vi "PH_Switch.ProcCases.vi"(0 "i ref in":refnum<vi>, 1 "selector":string, 2 "Data":T1, 3 "call cluster":T2={"Object"="", "Selector"="", "CallType"=enum."synchronous", "Async Object"="", "Async Selector"="", "Data Descriptor"="", "Data"=[], "Error #"=0, "Expire"=0}, 5 "error in (no error)":errorcluster) -> (14 "i ref out":refnum<vi>, 17 "answer cluster":T2={"Object"="", "Selector"="", "CallType"=enum."synchronous", "Async Object"="", "Async Selector"="", "Data Descriptor"="", "Data"=[], "Error #"=0, "Expire"=0}, 19 "error out":errorcluster)   [LabVIEW 2014, in "PH_Switch.lvlib"]
doc: "This method is called by a process from within the default case in the event loop. The methods of a class that are linked to events will be called from THIS method. Add your code here."
uses:
  PH_Switch.lvlib
  CSCore/CSSystem/CoreDefs/CoreDefs.call_type.ctl
  CSCore/BaseProcess/BaseProcess.descriptor string definition.ctl
  CSCore/CSSystem/CoreDefs/CoreDefs.rawDataType.ctl
  PH_StatusHandler/PH_StatusHandler.Status.ctl
  CSCore/CSSystem/CoreLib/CoreLib.string 2 byte array.vi
  CSCore/CSSystem/CoreLib/CoreLib.byte array 2 short.vi
  CSCore/CSSystem/CoreLib/CoreLib.byte array 2 string.vi
  PH_Common/PH_Common.lvlib
  CSCore/CSSystem/CoreLib/CoreLib.lvlib
  CSCore/BaseProcess/BaseProcess.lvlib
  CSCore/CAEObj/CAEObj.lvlib
  PH_Sixpack_Switch/PH_Sixpack_Switch.lvlib
  PH_PSDBWriter/PH_PSDBWriter.lvlib
  PH_StatusHandler/PH_StatusHandler.lvlib
  PH_Beckhoff/PH_Beckhoff.lvlib
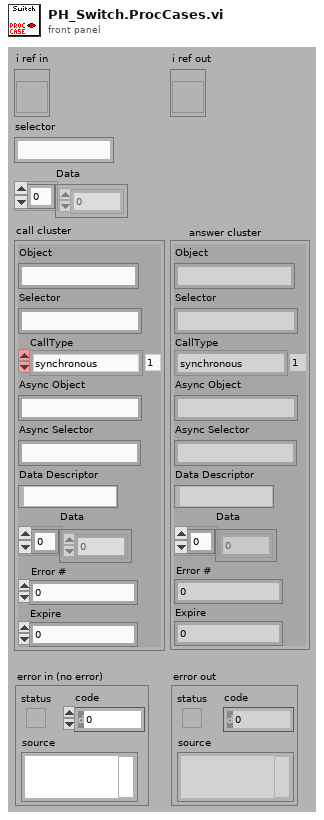
[diagram p1: front panel]
types:
  T1 = typedef "CoreDefs.rawDataType.ctl" = i8[]
  T2 = typedef "CoreDefs.call_type.ctl" = cluster{"Object":string, "Selector":string, "CallType":enum16{"simple", "synchronous", "asynchronous"}, "Async Object":string, "Async Selector":string, "Data Descriptor":T3, "Data":T1, "Error #":i32, "Expire":u32}
  T3 = typedef "BaseProcess.lvlib/BaseProcess.descriptor string definition.ctl" = string
  T4 = typedef "PH_Switch.lvlib/PH_Switch.i attribute.ctl" = cluster{"GUI Refs":T5, "Status true":T6, "Status false":T6, "Status Switch State":T6, "remote controlled":bool, "Tagname":cluster{"Switch":string, "True":string, "False":string}, "Beckhoff Instance":string, "Caption":cluster{"True":string, "False":string}, "Default State":string}
  T5 = typedef "PH_Switch.lvlib/PH_Switch.GUI Refs.ctl" = cluster{"true":refnum<vi>, "false":refnum<vi>, "Switch_state":refnum<vi>, "GUI-Knob":refnum<vi>, "Delete":refnum<vi>, "Function Textfield":refnum<vi>}
  T6 = typedef "PH_StatusHandler.lvlib/PH_StatusHandler.Status.ctl" = i16
  T7 = typedef "PH_PSDBWriter.lvlib/PH_PSDBWriter.PHELIX-Subsystems.ctl" = i32
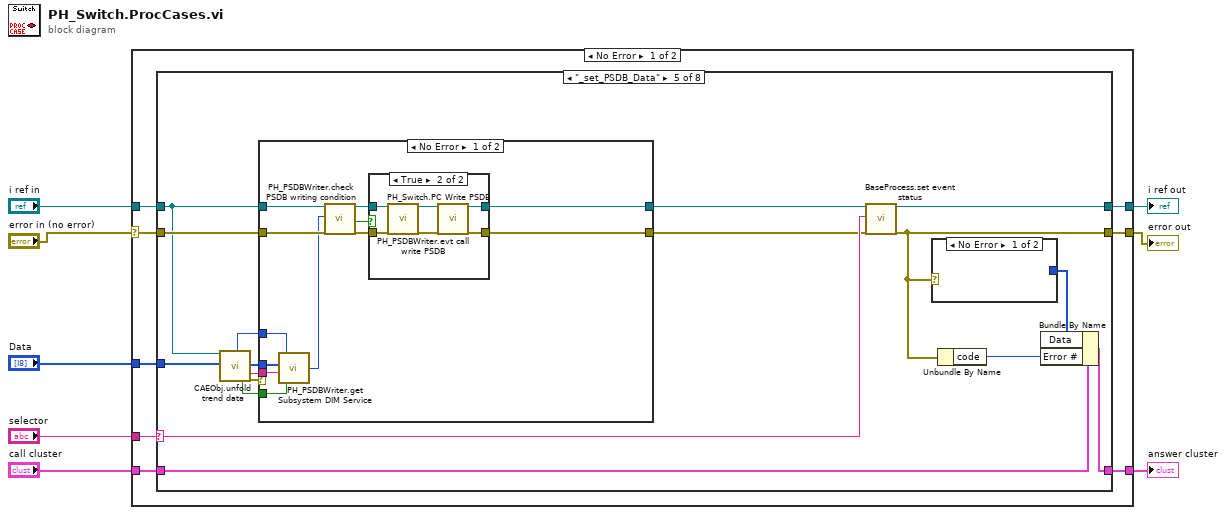
[diagram p0: block diagram]
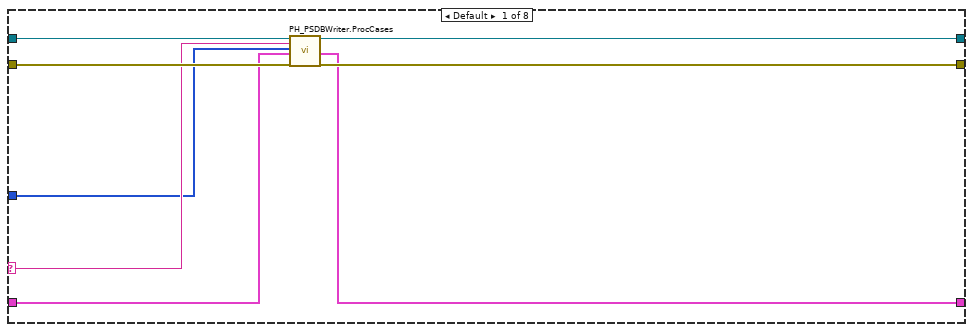
[diagram p2: hidden frame]
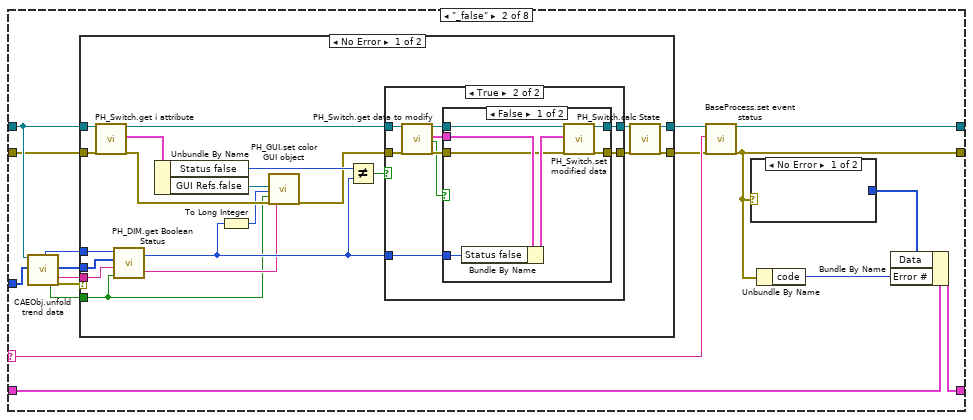
[diagram p3: hidden frame]
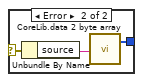
[diagram p7: hidden frame]
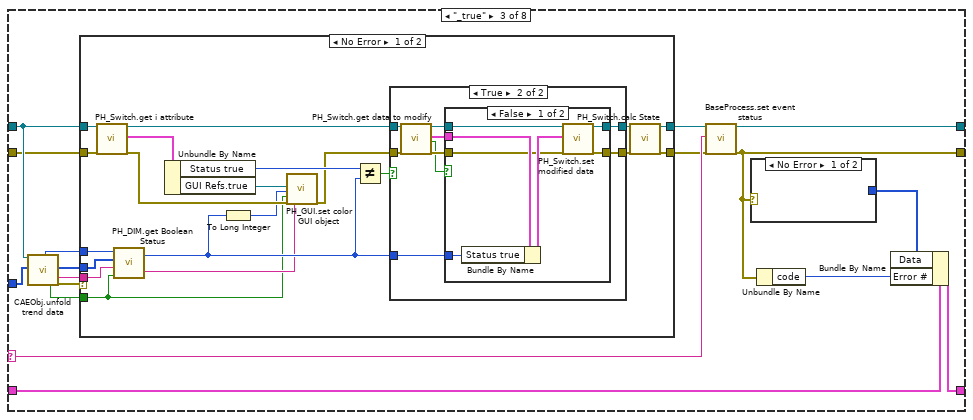
[diagram p8: hidden frame]
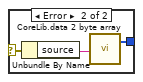
[diagram p12: hidden frame]
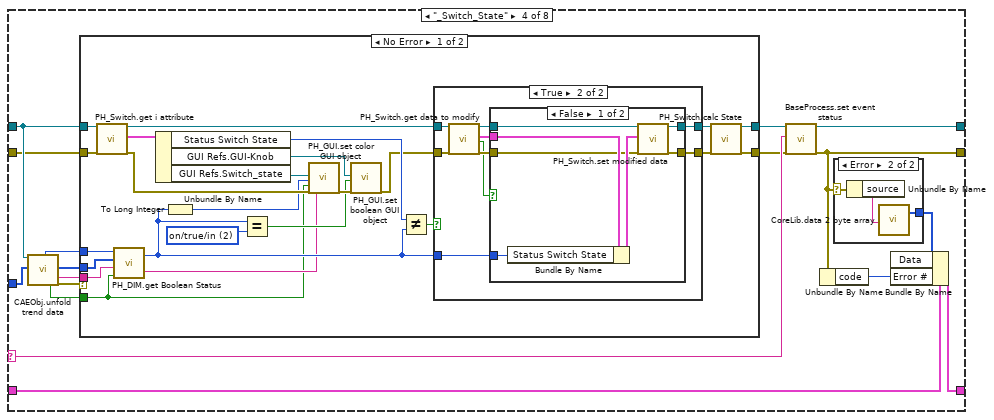
[diagram p13: hidden frame]
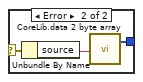
[diagram p20: hidden frame]
diagram:
  n1 = case shown="No Error" "error in (no error)" {
    selector: "error in (no error)" -> [w9 w383]
    tunnel: "selector" -> [w16 _]
    tunnel: [w15 w382] -> w7
    tunnel: "call cluster" -> [w14 w382]
    tunnel: "i ref in" -> [w13 w384]
    tunnel: [w12 w384] -> w5
    tunnel: [w11 w383] -> w4
    tunnel: "Data" -> [w10 _]
    frame No Error {
      n2 = case shown="\"_set_PSDB_Data\"" w16 {
        selector: w16 -> [w19 w39 w101 w163 w225 w261 w310 w353]
        tunnel: w13 -> [w18 w33 w95 w157 w216 w270 w314 w357]
        tunnel: [w24 w37 w99 w161 w228 w257 w312 w355] -> w12
        tunnel: w14 -> [w20 w35 w97 w159 w227 w260 w309 w352]
        tunnel: [w21 w34 w96 w158 w226 w259 w308 w351] -> w15
        tunnel: w9 -> [w23 w32 w94 w156 w219 w271 w313 w356]
        tunnel: [w22 w36 w98 w160 w229 w258 w311 w354] -> w11
        tunnel: w10 -> [w17 w38 w100 w162 w215 _ _ _]
        frame Default {
          n3 = call "PH_PSDBWriter.ProcCases.vi"("i ref in"=w18, "selector"=w19, "Data"=w17, "call cluster"=w20, "error in"=w23) -> ("i ref out"=w24:refnum<vi>, "answer cluster"=w21:T2, "error out"=w22:errorcluster)  [unwired: 12 in]
        }
        frame "_false" {
          n4 = call "CAEObj.unfold trend data.vi"("i ref in"=w33, "raw trend data"=w38) -> ("quality"=w26:i32, "no link"=w28:bool, "data"=w27:i8[], "typeDescriptor"=w25:string, "error out"=w29:errorcluster)  [unwired: 9 in, 4 out]
          n5 = case shown="No Error" w29 {
            tunnel: w32 -> [w61 w82]
            tunnel: [w52 w83] -> w30
            tunnel: [w50 w82] -> w31
            tunnel: w33 -> [w57 w83]
            tunnel: w28 -> [w42 _]
            tunnel: w25 -> [w60 _]
            tunnel: w27 -> [w58 _]
            tunnel: w26 -> [w59 _]
            frame No Error {
              n6 = call "PH_Switch.get i attribute.vi"("i ref in"=w57, "error in (no error)"=w61) -> ("i ref out"=w56:refnum<vi>, "i attribute"=w55:T4, "error out"=w47:errorcluster)  [unwired: 15 in]
              n7 = call "PH_DIM.get Boolean Status.vi"("no link"=w42, "typeDescriptor"=w60, "data"=w58, "quality"=w59) -> ("further information"=w44:string, "Status"=w45:T6)
              n8 = Unbundle By Name(w55) -> ("Status false"=w54:T6, "GUI Refs.false"=w48:refnum<vi>)
              n9 = To Long Integer(number=w45) -> (32bit integer=w43:i32)
              n10 = call "PH_GUI.set color GUI object.vi"("GUI object Ref"=w48, "State"=w43, "Blinking? (false)"=w42, "error in (no error)"=w47, "Tip Strip (N/A)"=w44) -> ("error out"=w46:errorcluster)  [unwired: 14 in]
              n11 = Not Equal?(x=w54, y=w45) -> (x != y?=w53:bool)
              n12 = case shown="True" w53 {
                tunnel: [w63 w65] -> w51
                tunnel: [w62 w64] -> w49
                tunnel: w46 -> [w62 w68]
                tunnel: w56 -> [w63 w67]
                tunnel: w45 -> [_ w66]
                frame False {
                }
                frame True {
                  n13 = call "PH_Switch.get data to modify.vi"("i ref in"=w67, "error in (no error)"=w68) -> ("i ref out"=w71:refnum<vi>, "i attribute"=w70:T4, "timed out"=w69:bool, "error out"=w72:errorcluster)  [unwired: 14 in]
                  n14 = case shown="False" w69 {
                    tunnel: w72 -> [w73 w81]
                    tunnel: [w79 w81] -> w64
                    tunnel: [w78 w80] -> w65
                    tunnel: w71 -> [w74 w80]
                    tunnel: w70 -> [w77 _]
                    tunnel: w66 -> [w75 _]
                    frame False {
                      n15 = Bundle By Name(cluster=w77, "Status false"=w75) -> (w76:T4)
                      n16 = call "PH_Switch.set modified data.vi"("i ref in"=w74, "i attribute"=w76, "error in (no error)"=w73) -> ("i ref out"=w78:refnum<vi>, "error out"=w79:errorcluster)  [unwired: 15 in]
                    }
                    frame True {
                    }
                  }
                }
              }
              n17 = call "PH_Switch.calc State.vi"("i ref in"=w51, "error in (no error)"=w49) -> ("i ref out"=w52:refnum<vi>, "error out"=w50:errorcluster)  [unwired: 16 in]
            }
            frame Error {
            }
          }
          n18 = call "BaseProcess.set event status.vi"("i ref in"=w30, "EventStatus"=w39, "error in (no error)"=w31) -> ("i ref out"=w37:refnum<vi>, "error out"=w36:errorcluster)  [unwired: 14 in, 1 out]
          n19 = case shown="No Error" w36 {
            selector: w36 -> [_ w86]
            tunnel: [_ w84] -> w41
            frame No Error {
            }
            frame Error {
              n20 = Unbundle By Name(w86) -> ("source"=w85:string)
              n21 = call-poly "CoreLib.data 2 byte array.vi"("string"=w85) -> ("byteArray out"=w84:T1)  [unwired: 18 in]
            }
          }
          n22 = Unbundle By Name(w36) -> ("code"=w40:i32)
          n23 = Bundle By Name(cluster=w35, "Data"=w41, "Error #"=w40) -> (w34:T2)
        }
        frame "_true" {
          n24 = call "CAEObj.unfold trend data.vi"("i ref in"=w95, "raw trend data"=w100) -> ("quality"=w88:i32, "no link"=w90:bool, "data"=w89:i8[], "typeDescriptor"=w87:string, "error out"=w91:errorcluster)  [unwired: 9 in, 4 out]
          n25 = case shown="No Error" w91 {
            tunnel: w94 -> [w123 w144]
            tunnel: [w113 w145] -> w92
            tunnel: [w111 w144] -> w93
            tunnel: w95 -> [w119 w145]
            tunnel: w90 -> [w104 _]
            tunnel: w87 -> [w122 _]
            tunnel: w89 -> [w120 _]
            tunnel: w88 -> [w121 _]
            frame No Error {
              n26 = call "PH_Switch.get i attribute.vi"("i ref in"=w119, "error in (no error)"=w123) -> ("i ref out"=w118:refnum<vi>, "i attribute"=w117:T4, "error out"=w109:errorcluster)  [unwired: 15 in]
              n27 = call "PH_DIM.get Boolean Status.vi"("no link"=w104, "typeDescriptor"=w122, "data"=w120, "quality"=w121) -> ("further information"=w105:string, "Status"=w107:T6)
              n28 = Unbundle By Name(w117) -> ("Status true"=w116:T6, "GUI Refs.true"=w110:refnum<vi>)
              n29 = To Long Integer(number=w107) -> (32bit integer=w106:i32)
              n30 = call "PH_GUI.set color GUI object.vi"("GUI object Ref"=w110, "State"=w106, "Blinking? (false)"=w104, "error in (no error)"=w109, "Tip Strip (N/A)"=w105) -> ("error out"=w108:errorcluster)  [unwired: 14 in]
              n31 = Not Equal?(x=w116, y=w107) -> (x != y?=w115:bool)
              n32 = case shown="True" w115 {
                tunnel: [w125 w127] -> w112
                tunnel: [w124 w126] -> w114
                tunnel: w108 -> [w124 w130]
                tunnel: w118 -> [w125 w129]
                tunnel: w107 -> [_ w128]
                frame False {
                }
                frame True {
                  n33 = call "PH_Switch.get data to modify.vi"("i ref in"=w129, "error in (no error)"=w130) -> ("i ref out"=w133:refnum<vi>, "i attribute"=w132:T4, "timed out"=w131:bool, "error out"=w134:errorcluster)  [unwired: 14 in]
                  n34 = case shown="False" w131 {
                    tunnel: w134 -> [w135 w143]
                    tunnel: [w141 w143] -> w126
                    tunnel: [w140 w142] -> w127
                    tunnel: w133 -> [w136 w142]
                    tunnel: w132 -> [w139 _]
                    tunnel: w128 -> [w137 _]
                    frame False {
                      n35 = Bundle By Name(cluster=w139, "Status true"=w137) -> (w138:T4)
                      n36 = call "PH_Switch.set modified data.vi"("i ref in"=w136, "i attribute"=w138, "error in (no error)"=w135) -> ("i ref out"=w140:refnum<vi>, "error out"=w141:errorcluster)  [unwired: 15 in]
                    }
                    frame True {
                    }
                  }
                }
              }
              n37 = call "PH_Switch.calc State.vi"("i ref in"=w112, "error in (no error)"=w114) -> ("i ref out"=w113:refnum<vi>, "error out"=w111:errorcluster)  [unwired: 16 in]
            }
            frame Error {
            }
          }
          n38 = call "BaseProcess.set event status.vi"("i ref in"=w92, "EventStatus"=w101, "error in (no error)"=w93) -> ("i ref out"=w99:refnum<vi>, "error out"=w98:errorcluster)  [unwired: 14 in, 1 out]
          n39 = case shown="No Error" w98 {
            selector: w98 -> [_ w148]
            tunnel: [_ w146] -> w103
            frame No Error {
            }
            frame Error {
              n40 = Unbundle By Name(w148) -> ("source"=w147:string)
              n41 = call-poly "CoreLib.data 2 byte array.vi"("string"=w147) -> ("byteArray out"=w146:T1)  [unwired: 18 in]
            }
          }
          n42 = Unbundle By Name(w98) -> ("code"=w102:i32)
          n43 = Bundle By Name(cluster=w97, "Data"=w103, "Error #"=w102) -> (w96:T2)
        }
        frame "_Switch_State" {
          n44 = call "CAEObj.unfold trend data.vi"("i ref in"=w157, "raw trend data"=w162) -> ("quality"=w150:i32, "no link"=w152:bool, "data"=w151:i8[], "typeDescriptor"=w149:string, "error out"=w153:errorcluster)  [unwired: 9 in, 4 out]
          n45 = case shown="No Error" w153 {
            tunnel: w156 -> [w189 w210]
            tunnel: [w178 w211] -> w154
            tunnel: [w177 w210] -> w155
            tunnel: w157 -> [w185 w211]
            tunnel: w152 -> [w166 _]
            tunnel: w149 -> [w188 _]
            tunnel: w151 -> [w186 _]
            tunnel: w150 -> [w187 _]
            frame No Error {
              w168 = T6 2 items=["no info", "off/false/out", "on/true/in", "Failure", "Alarm", "Status 1", "Status 2", "Status 3"] ("y")
              n46 = call "PH_Switch.get i attribute.vi"("i ref in"=w185, "error in (no error)"=w189) -> ("i ref out"=w184:refnum<vi>, "i attribute"=w183:T4, "error out"=w175:errorcluster)  [unwired: 15 in]
              n47 = call "PH_DIM.get Boolean Status.vi"("no link"=w166, "typeDescriptor"=w188, "data"=w186, "quality"=w187) -> ("further information"=w167:string, "Status"=w170:T6)
              n48 = Unbundle By Name(w183) -> ("Status Switch State"=w182:T6, "GUI Refs.GUI-Knob"=w172:refnum<vi>, "GUI Refs.Switch_state"=w173:refnum<vi>)
              n49 = To Long Integer(number=w170) -> (32bit integer=w169:i32)
              n50 = Equal?(x=w170, y=w168) -> (x = y?=w171:bool)
              n51 = call "PH_GUI.set color GUI object.vi"("GUI object Ref"=w173, "State"=w169, "Blinking? (false)"=w166, "error in (no error)"=w175, "Tip Strip (N/A)"=w167) -> ("error out"=w176:errorcluster)  [unwired: 14 in]
              n52 = call "PH_GUI.set boolean GUI object.vi"("Boolean Knob GUI Ref"=w172, "Value"=w171, "error in (no error)"=w176) -> ("error out"=w174:errorcluster)  [unwired: 16 in]
              n53 = Not Equal?(x=w182, y=w170) -> (x != y?=w181:bool)
              n54 = case shown="True" w181 {
                tunnel: [w191 w193] -> w180
                tunnel: [w190 w192] -> w179
                tunnel: w174 -> [w190 w196]
                tunnel: w184 -> [w191 w195]
                tunnel: w170 -> [_ w194]
                frame False {
                }
                frame True {
                  n55 = call "PH_Switch.get data to modify.vi"("i ref in"=w195, "error in (no error)"=w196) -> ("i ref out"=w199:refnum<vi>, "i attribute"=w198:T4, "timed out"=w197:bool, "error out"=w200:errorcluster)  [unwired: 14 in]
                  n56 = case shown="False" w197 {
                    tunnel: w200 -> [w201 w209]
                    tunnel: [w207 w209] -> w192
                    tunnel: [w206 w208] -> w193
                    tunnel: w199 -> [w203 w208]
                    tunnel: w198 -> [w205 _]
                    tunnel: w194 -> [w202 _]
                    frame False {
                      n57 = Bundle By Name(cluster=w205, "Status Switch State"=w202) -> (w204:T4)
                      n58 = call "PH_Switch.set modified data.vi"("i ref in"=w203, "i attribute"=w204, "error in (no error)"=w201) -> ("i ref out"=w206:refnum<vi>, "error out"=w207:errorcluster)  [unwired: 15 in]
                    }
                    frame True {
                    }
                  }
                }
              }
              n59 = call "PH_Switch.calc State.vi"("i ref in"=w180, "error in (no error)"=w179) -> ("i ref out"=w178:refnum<vi>, "error out"=w177:errorcluster)  [unwired: 16 in]
            }
            frame Error {
            }
          }
          n60 = call "BaseProcess.set event status.vi"("i ref in"=w154, "EventStatus"=w163, "error in (no error)"=w155) -> ("i ref out"=w161:refnum<vi>, "error out"=w160:errorcluster)  [unwired: 14 in, 1 out]
          n61 = Unbundle By Name(w160) -> ("code"=w164:i32)
          n62 = case shown="Error" w160 {
            selector: w160 -> [_ w214]
            tunnel: [_ w212] -> w165
            frame No Error {
            }
            frame Error {
              n63 = Unbundle By Name(w214) -> ("source"=w213:string)
              n64 = call-poly "CoreLib.data 2 byte array.vi"("string"=w213) -> ("byteArray out"=w212:T1)  [unwired: 18 in]
            }
          }
          n65 = Bundle By Name(cluster=w159, "Data"=w165, "Error #"=w164) -> (w158:T2)
        }
        frame "_set_PSDB_Data" {
          n66 = call "CAEObj.unfold trend data.vi"("i ref in"=w216, "raw trend data"=w215) -> ("quality"=w222:i32, "no link"=w221:bool, "data"=w224:i8[], "typeDescriptor"=w223:string, "error out"=w220:errorcluster)  [unwired: 9 in, 4 out]
          n67 = case shown="No Error" w220 {
            tunnel: w219 -> [w243 w253]
            tunnel: [w242 w252] -> w218
            tunnel: [w241 w253] -> w217
            tunnel: w216 -> [w235 w252]
            tunnel: w221 -> [w240 _]
            tunnel: w223 -> [w239 _]
            tunnel: w224 -> [w238 _]
            tunnel: w222 -> [w237 _]
            frame No Error {
              n68 = call "PH_PSDBWriter.get Subsystem DIM Service.vi"("no link"=w240, "typeDescriptor"=w239, "data"=w238, "quality"=w237) -> ("PHELIX Subsystems"=w232:T7)
              n69 = call "PH_PSDBWriter.check PSDB writing condition.vi"("i ref in"=w235, "wanted Subsystem"=w232, "error IO"=w243) -> ("i ref out"=w234:refnum<vi>, "write PSDB?"=w233:bool, "error out"=w236:errorcluster)  [unwired: 14 in]
              n70 = case shown="True" w233 {
                tunnel: w236 -> [w244 w251]
                tunnel: [w245 w246] -> w242
                tunnel: [w244 w247] -> w241
                tunnel: w234 -> [w245 w250]
                frame False {
                }
                frame True {
                  n71 = call "PH_Switch.PC Write PSDB.vi"("i ref in"=w250, "error IO"=w251) -> ("i ref out"=w249:refnum<vi>, "error out"=w248:errorcluster)  [unwired: 16 in]
                  n72 = call "PH_PSDBWriter.evt call write PSDB.vi"("i ref in"=w249, "error in (no error)"=w248) -> ("i ref out"=w246:refnum<vi>, "error out"=w247:errorcluster)  [unwired: 16 in]
                }
              }
            }
            frame Error {
            }
          }
          n73 = call "BaseProcess.set event status.vi"("i ref in"=w218, "EventStatus"=w225, "error in (no error)"=w217) -> ("i ref out"=w228:refnum<vi>, "error out"=w229:errorcluster)  [unwired: 14 in, 1 out]
          n74 = case shown="No Error" w229 {
            selector: w229 -> [_ w256]
            tunnel: [_ w254] -> w230
            frame No Error {
            }
            frame Error {
              n75 = Unbundle By Name(w256) -> ("source"=w255:string)
              n76 = call-poly "CoreLib.data 2 byte array.vi"("string"=w255) -> ("byteArray out"=w254:T1)  [unwired: 18 in]
            }
          }
          n77 = Unbundle By Name(w229) -> ("code"=w231:i32)
          n78 = Bundle By Name(cluster=w227, "Data"=w230, "Error #"=w231) -> (w226:T2)
        }
        frame "Switch" {
          n79 = Unbundle By Name(w260) -> ("Data"=w269:T1)
          n80 = call-poly "CoreLib.byte array 2 data.vi"("byteArray"=w269) -> ("i16"=w268:i16, "error out"=w267:errorcluster)  [unwired: 16 in, 1 out]
          n81 = Greater Than 0?(x=w268) -> (x > 0?=w266:bool)
          n82 = case shown="No Error" w267 {
            tunnel: [w284 w307] -> w263
            tunnel: [w283 w304] -> w262
            tunnel: w270 -> [w277 w307]
            tunnel: w271 -> [w276 w306]
            tunnel: w261 -> [_ w305]
            tunnel: w266 -> [w282 _]
            frame No Error {
              n83 = call "PH_Switch.get i attribute.vi"("i ref in"=w277, "error in (no error)"=w276) -> ("i ref out"=w285:refnum<vi>, "i attribute"=w287:T4, "error out"=w286:errorcluster)  [unwired: 15 in]
              n84 = Unbundle By Name(w287) -> ("GUI Refs.GUI-Knob"=w280:refnum<vi>, "Beckhoff Instance"=w278:string, "Tagname.Switch"=w275:string)
              n85 = call "PH_Switch.check 6P Switch.vi"("Tagname"=w275) -> ("Tagname 6P Switch"=w281:string, "6P Switch?"=w279:bool)
              n86 = case shown="False" w279 {
                tunnel: w286 -> [w294 w303]
                tunnel: w285 -> [w296 w302]
                tunnel: [w295 w301] -> w284
                tunnel: [w290 w300] -> w283
                tunnel: w278 -> [_ w299]
                tunnel: w282 -> [w292 w298]
                tunnel: w275 -> [_ w297]
                tunnel: w281 -> [w293 _]
                tunnel: w280 -> [w289 _]
                frame True {
                  n87 = call "PH_Sixpack_Switch.evt move.vi"("i ref in"=w296, "Instance"=w293, "Move"=w292, "error in (no error)"=w294) -> ("i ref out"=w295:refnum<vi>, "error out"=w291:errorcluster)  [unwired: 14 in]
                  n88 = call "PH_GUI.set boolean GUI object.vi"("Boolean Knob GUI Ref"=w289, "Value"=FALSE, "error in (no error)"=w291) -> ("error out"=w290:errorcluster)  [unwired: 16 in]
                }
                frame False {
                  n89 = call "PH_Beckhoff.evt Call Set Boolean Value.vi"("i ref in"=w302, "Beckhoff Instance"=w299, "Tagname to set"=w297, "Value"=w298, "error in"=w303) -> ("i ref out"=w301:refnum<vi>, "error out"=w300:errorcluster)  [unwired: 13 in]
                }
              }
            }
            frame Error {
              n90 = call "CoreLib.set data type mismatch.vi"("error in (no error)"=w306, "error source"=w305) -> ("error out"=w304:errorcluster)  [unwired: 17 in]
            }
          }
          n91 = call "BaseProcess.set event status.vi"("i ref in"=w263, "EventStatus"=w261, "error in (no error)"=w262) -> ("i ref out"=w257:refnum<vi>, "error out"=w258:errorcluster)  [unwired: 14 in, 1 out]
          n92 = Unbundle By Name(w258) -> ("code"=w265:i32)
          n93 = case shown="No Error" w258 {
            selector: w258 -> [_ w274]
            tunnel: [_ w272] -> w264
            frame No Error {
            }
            frame Error {
              n94 = Unbundle By Name(w274) -> ("source"=w273:string)
              n95 = call-poly "CoreLib.data 2 byte array.vi"("string"=w273) -> ("byteArray out"=w272:T1)  [unwired: 18 in]
            }
          }
          n96 = Bundle By Name(cluster=w260, "Data"=w264, "Error #"=w265) -> (w259:T2)
        }
        frame "Control Remote" {
          n97 = Unbundle By Name(w309) -> ("Data"=w317:T1)
          n98 = call-poly "CoreLib.byte array 2 data.vi"("byteArray"=w317) -> ("i16"=w318:i16, "error out"=w320:errorcluster)  [unwired: 16 in, 1 out]
          n99 = Greater Than 0?(x=w318) -> (x > 0?=w319:bool)
          n100 = case shown="No Error" w320 {
            tunnel: [w329 w349] -> w315
            tunnel: w314 -> [w336 w349]
            tunnel: w313 -> [w335 w348]
            tunnel: [w327 w347] -> w316
            tunnel: w310 -> [_ w346]
            tunnel: w319 -> [w333 _]
            frame No Error {
              n101 = call "PH_Switch.get data to modify.vi"("i ref in"=w336, "error in (no error)"=w335) -> ("i ref out"=w331:refnum<vi>, "i attribute"=w332:T4, "timed out"=w330:bool, "error out"=w334:errorcluster)  [unwired: 14 in]
              n102 = case shown="False" w330 {
                tunnel: w334 -> [w343 w345]
                tunnel: [w342 w345] -> w326
                tunnel: w333 -> [w337 _]
                tunnel: w332 -> [w341 _]
                tunnel: w331 -> [w340 w344]
                tunnel: [w339 w344] -> w328
                frame False {
                  n103 = Bundle By Name(cluster=w341, "remote controlled"=w337) -> (w338:T4)
                  n104 = call "PH_Switch.set modified data.vi"("i ref in"=w340, "i attribute"=w338, "error in (no error)"=w343) -> ("i ref out"=w339:refnum<vi>, "error out"=w342:errorcluster)  [unwired: 15 in]
                }
                frame True {
                }
              }
              n105 = call "PH_Switch.calc State.vi"("i ref in"=w328, "error in (no error)"=w326) -> ("i ref out"=w329:refnum<vi>, "error out"=w327:errorcluster)  [unwired: 16 in]
            }
            frame Error {
              n106 = call "CoreLib.set data type mismatch.vi"("error in (no error)"=w348, "error source"=w346) -> ("error out"=w347:errorcluster)  [unwired: 17 in]
            }
          }
          n107 = call "BaseProcess.set event status.vi"("i ref in"=w315, "EventStatus"=w310, "error in (no error)"=w316) -> ("i ref out"=w312:refnum<vi>, "error out"=w311:errorcluster)  [unwired: 14 in, 1 out]
          n108 = case shown="Error" w311 {
            selector: w311 -> [_ w325]
            tunnel: [_ w323] -> w322
            frame No Error {
            }
            frame Error {
              n109 = Unbundle By Name(w325) -> ("source"=w324:string)
              n110 = call-poly "CoreLib.data 2 byte array.vi"("string"=w324) -> ("byteArray out"=w323:T1)  [unwired: 18 in]
            }
          }
          n111 = Unbundle By Name(w311) -> ("code"=w321:i32)
          n112 = Bundle By Name(cluster=w309, "Data"=w322, "Error #"=w321) -> (w308:T2)
        }
        frame "Set Function Textfield" {
          n113 = Unbundle By Name(w352) -> ("Data"=w360:T1)
          n114 = call-poly "CoreLib.byte array 2 data.vi"("byteArray"=w360) -> ("string"=w350:string, "error out"=w361:errorcluster)  [unwired: 16 in, 1 out]
          n115 = case shown="No Error" w361 {
            tunnel: [w373 w381] -> w358
            tunnel: w357 -> [w375 w381]
            tunnel: w356 -> [w374 w380]
            tunnel: [w371 w379] -> w359
            tunnel: w353 -> [_ w378]
            tunnel: w350 -> [w368 _]
            frame No Error {
              n116 = call "PH_Switch.get i attribute.vi"("i ref in"=w375, "error in (no error)"=w374) -> ("i ref out"=w373:refnum<vi>, "i attribute"=w370:T4, "error out"=w372:errorcluster)  [unwired: 15 in]
              n117 = Unbundle By Name(w370) -> ("GUI Refs.Function Textfield"=w369:refnum<vi>)
              n118 = case shown="\"\", \"N/A\"" w368 {
                tunnel: [TRUE FALSE] -> w367
                frame Default {
                }
                frame "", "N/A" {
                }
              }
              n119 = call "PH_GUI.set string GUI object.vi"("Visible (True)"=w367, "GUI object Ref"=w369, "Text"=w368, "error in"=w372) -> ("error out"=w371:errorcluster)  [unwired: 15 in]
            }
            frame Error {
              n120 = call "CoreLib.set data type mismatch.vi"("error in (no error)"=w380, "error source"=w378) -> ("error out"=w379:errorcluster)  [unwired: 17 in]
            }
          }
          n121 = call "BaseProcess.set event status.vi"("i ref in"=w358, "EventStatus"=w353, "error in (no error)"=w359) -> ("i ref out"=w355:refnum<vi>, "error out"=w354:errorcluster)  [unwired: 14 in, 1 out]
          n122 = case shown="Error" w354 {
            selector: w354 -> [_ w366]
            tunnel: [_ w364] -> w363
            frame No Error {
            }
            frame Error {
              n123 = Unbundle By Name(w366) -> ("source"=w365:string)
              n124 = call-poly "CoreLib.data 2 byte array.vi"("string"=w365) -> ("byteArray out"=w364:T1)  [unwired: 18 in]
            }
          }
          n125 = Unbundle By Name(w354) -> ("code"=w362:i32)
          n126 = Bundle By Name(cluster=w352, "Data"=w363, "Error #"=w362) -> (w351:T2)
        }
      }
    }
    frame Error {
    }
  }
  "answer cluster" <- w7
  "i ref out" <- w5
  "error out" <- w4
